vi "Write.vi"(8 "error in":errorcluster, 9 "Data":u8[](array[numeric]) format="%.0x", 10 "CAN-ID":u32 format="%.0x", 11 "CANopen in":refnum<class "CANopen.lvclass">) -> (0 "error out":errorcluster, 3 "CANopen out":refnum<class "CANopen.lvclass">)   [LabVIEW 2024, in "canopen.lvlib" / "CANopen.lvclass"]
doc: "Sends a bunch of data to a specific COB-ID."
uses:
  CANopen.lvclass
  CANopen.lvclass/CANopen.ctl
  HAL/HAL/Protocols/ICAN/ICAN.lvclass
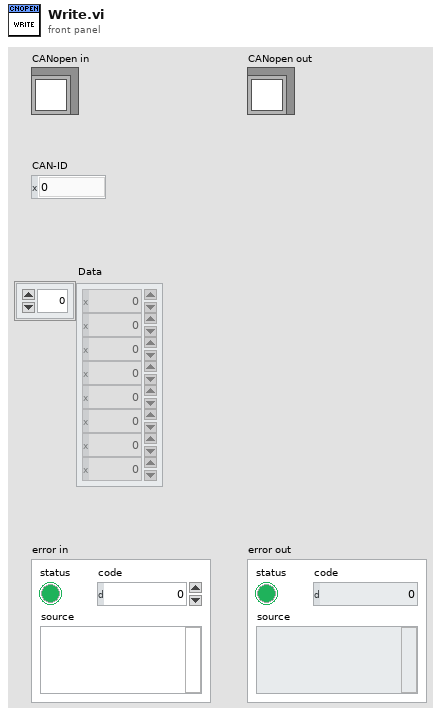
[diagram p1: front panel]
types:
  T1 = cluster{"ID":u32, "MSG type":u8, "DLC":u8, "DATA":u8[]}
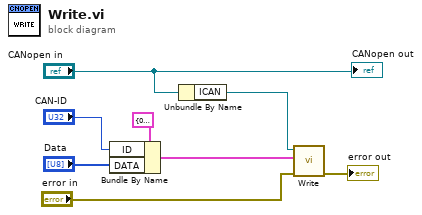
[diagram p0: block diagram]
diagram:
  n1 = Bundle By Name(cluster=T1 {"ID"=0, "MSG type"=0, "DLC"=0, "DATA"=[]} ("CAN Message"), "ID"="CAN-ID", "DATA"="Data") -> (w7:T1)
  n2 = Unbundle By Name("CANopen in") -> ("ICAN"=w6:refnum<class "ICAN.lvclass">)
  n3 = call-dynamic "Write.vi"("error in"="error in", "CAN Message"=w7, "ICAN in"=w6) -> ("error out"=→"error out":errorcluster)  [unwired: 7 in, 1 out]
  "CANopen out" <- "CANopen in"
